vi "Write Relay Count.vi"(8 "error in (no error)":errorcluster, 10 "Relay Count":i32, 11 "Route Manager in":refnum<class "Route Manager.lvclass">) -> (0 "error out":errorcluster, 3 "Route Manager out":refnum<class "Route Manager.lvclass">)   [LabVIEW 2015, in "Route Manager.lvclass"]
uses:
  Route Manager.lvclass
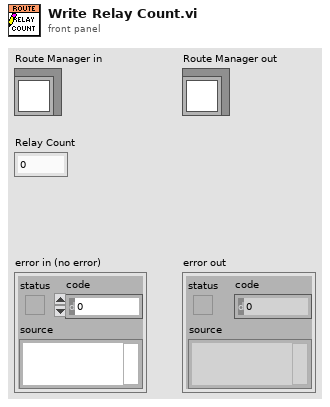
[diagram p1: front panel]
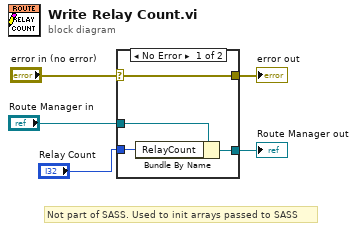
[diagram p0: block diagram]
diagram:
  # "Not part of SASS. Used to init arrays passed to SASS"
  n1 = case shown="No Error" "error in (no error)" {
    selector: "error in (no error)" -> [w9 w10]
    tunnel: [w9 w10] -> w4
    tunnel: [w7 w11] -> w2
    tunnel: "Route Manager in" -> [w8 w11]
    tunnel: "Relay Count" -> [w6 _]
    frame No Error {
      n2 = Bundle By Name(cluster=w8, "RelayCount"=w6) -> (w7:refnum<class "Route Manager.lvclass">)
    }
    frame Error {
    }
  }
  "error out" <- w4
  "Route Manager out" <- w2
